vi "move.vi"(0 "walls/field":T2[][](array[typedef]), 2 "direction":T3 items=["^", "^>", ">", "V>", "V", "<V", "<", "<^"], 3 "Drone":T1) -> (6 "walls/field":T2[][](array[typedef]), 9 "Drone":T1)   [LabVIEW 2009]
uses:
  direction.ctl
  square.ctl
  Drone data.ctl
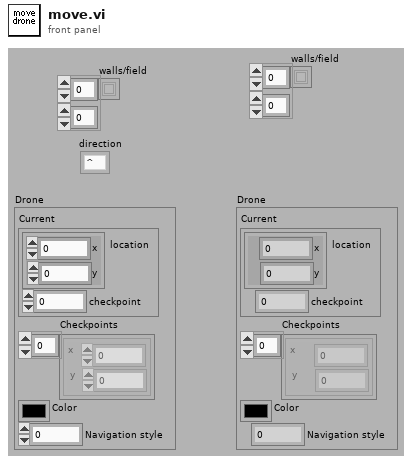
[diagram p1: front panel]
types:
  T1 = typedef "Drone data.ctl" = cluster{"Current":cluster{"location":cluster{"x":i16, "y":i16}, "checkpoint":i32}, "Checkpoints":cluster{"x":i16, "y":i16}[], "Color":u32, "Navigation style":i32}
  T2 = typedef "square.ctl" = u8
  T3 = typedef "direction.ctl" = i8
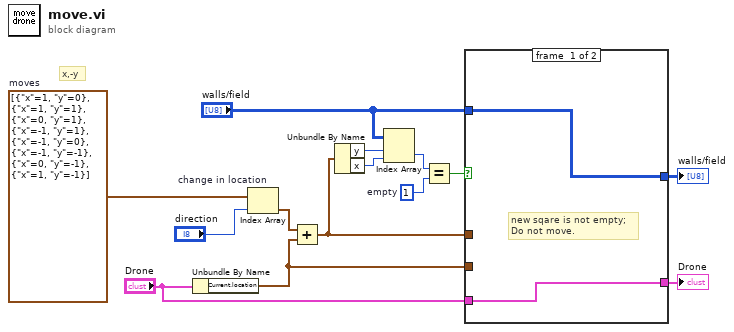
[diagram p0: block diagram]
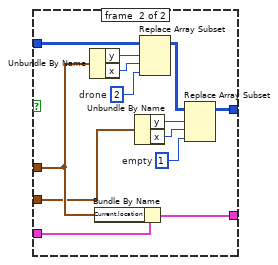
[diagram p2: hidden frame]
diagram:
  w8 = T2 1  # empty
  w14 = cluster{"x":i16, "y":i16}[] [{"x"=1, "y"=0}, {"x"=1, "y"=1}, {"x"=0, "y"=1}, {"x"=-1, "y"=1}, {"x"=-1, "y"=0}, {"x"=-1, "y"=-1}, {"x"=0, "y"=-1}, {"x"=1, "y"=-1}]  # moves
  # "x,-y"
  n1 = Unbundle By Name("Drone") -> ("Current.location"=w5:cluster{"x":i16, "y":i16})
  n2 = Index Array "change in location"(array=w14, index="direction") -> (element=w12:cluster{"x":i16, "y":i16})
  n3 = Add(x=w12, y=w5) -> (x+y=w6:cluster{"x":i16, "y":i16})
  n4 = Unbundle By Name(w6) -> ("y"=w11:i16, "x"=w10:i16)
  n5 = Index Array(array="walls/field", index (row)=w11, index (col)=w10) -> (element=w9:T2)
  n6 = Equal?(x=w9, y=w8) -> (x = y?=w7:bool)
  n7 = case shown="True" w7 {
    tunnel: w6 -> [_ w26]
    tunnel: w5 -> [_ w18]
    tunnel: "Drone" -> [w16 w29]
    tunnel: [w16 w28] -> w1
    tunnel: "walls/field" -> [w15 w27]
    tunnel: [w15 w17] -> w2
    frame #0 {
      # "new sqare is not empty;\nDo not move."
    }
    frame #1 {
      w22 = T2 1  # empty
      w23 = T2 2  # drone
      n8 = Unbundle By Name(w26) -> ("y"=w24:i16, "x"=w25:i16)
      n9 = Bundle By Name(cluster=w29, "Current.location"=w26) -> (w28:T1)
      n10 = Unbundle By Name(w18) -> ("y"=w21:i16, "x"=w20:i16)
      n11 = Replace Array Subset(array=w27, new element=w23, index (row)=w24, index (col)=w25) -> (w19:T2[][])
      n12 = Replace Array Subset(array=w19, new element=w22, index (row)=w21, index (col)=w20) -> (w17:T2[][])
    }
  }
  "walls/field" <- w2
  "Drone" <- w1
